vi "From 2D Float Tree Data.vi"(11 "Tree Data":refnum<class "Tree Data.lvclass">) -> (2 "2D Flt":dbl[][](array[numeric]))   [LabVIEW 2020, in "NI_VIAnCFGDataStructure.lvlib" / "2D Flt.lvclass"]
doc: "Extract a 2D Float value from Tree Data type."
uses:
  <vilib>/addons/analyzer/VIAnCFGDataStructure/Data Types/2D Flt/2D Flt.lvclass
  <vilib>/addons/analyzer/VIAnCFGDataStructure/Tree Data/Tree Data.lvclass
  <vilib>/addons/analyzer/VIAnCFGDataStructure/Data Types/2D Flt/2D Flt.lvclass/2D Flt.ctl
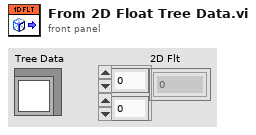
[diagram p1: front panel]
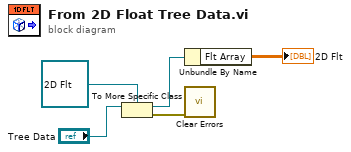
[diagram p0: block diagram]
diagram:
  n1 = To More Specific Class(target class=refnum<class "2D Flt.lvclass"> refnum ("Tree API.lvlib:2D Flt.lvclass"), reference="Tree Data") -> (specific class reference=w4:refnum<class "2D Flt.lvclass">, error out=w3:errorcluster)  [unwired: 1 in]
  n2 = Unbundle By Name(w4) -> ("Flt Array"=→"2D Flt":dbl[][])
  n3 = call <vilib>:"Clear Errors.vi"("error in (no error)"=w3) -> ()  [unwired: 5 in, 2 out]
